vi "Comp-HorarioSeg.vi"(1 "Lower limit":string, 2 "Upper limit":string) -> (0 "In Range?":bool)   [LabVIEW 2012]
panel:
  out "S string":string
  out "M string":string
  out "H string":string
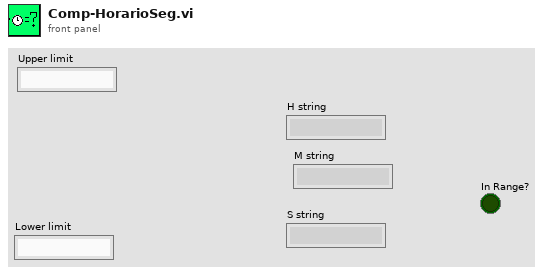
[diagram p1: front panel]
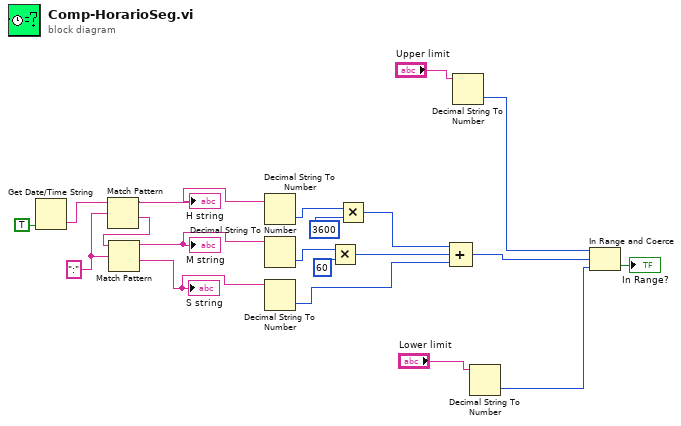
[diagram p0: block diagram]
diagram:
  w14 = ":" ("search string/char (-)")
  n1 = Get Date/Time String(want seconds? (F)=TRUE) -> (time string=w16:string)  [unwired: 2 in, 1 out]
  n2 = Match Pattern(string=w16, regular expression=w14) -> (before substring=w13:string, after substring=w15:string)  [unwired: 1 in, 2 out]
  "H string" <- w13
  n3 = Match Pattern(string=w15, regular expression=w14) -> (before substring=w12:string, after substring=w11:string)  [unwired: 1 in, 2 out]
  "M string" <- w12
  "S string" <- w11
  n4 = Decimal String To Number(string=w13) -> (number=w7:i32)  [unwired: 2 in, 1 out]
  n5 = Decimal String To Number(string=w12) -> (number=w8:i32)  [unwired: 2 in, 1 out]
  n6 = Decimal String To Number(string=w11) -> (number=w4:i32)  [unwired: 2 in, 1 out]
  n7 = Multiply(x=w8, y=60 ("offset past number")) -> (x*y=w5:i32)
  n8 = Multiply(x=w7, y=3600 ("offset past number")) -> (x*y=w6:i32)
  n9 = Compound Arithmetic op=ADD(w6, w5, w4) -> (w18:i32)
  n10 = Decimal String To Number(string="Upper limit") -> (number=w3:i32)  [unwired: 2 in, 1 out]
  n11 = Decimal String To Number(string="Lower limit") -> (number=w1:i32)  [unwired: 2 in, 1 out]
  n12 = In Range and Coerce(upper limit=w3, x=w18, lower limit=w1) -> (In Range?=→"In Range?":bool)  [unwired: 1 out]
